vi "Pre Launch Init.vi"(11 "Nested in":refnum<class "MDI Panel Actor.lvclass">) -> (0 "error out":errorcluster, 3 "Nested out":refnum<class "MDI Panel Actor.lvclass">)   [LabVIEW 2018, in "MDI Panel Actor.lvlib" / "MDI Panel Actor.lvclass"]
uses:
  MDI Panel Actor.lvclass
  MDI Panel Actor.lvclass/MDI Panel Actor.ctl
  <vilib>/MGI/Panel Manager/Panel Actor/Panel Actor/Panel Actor.lvclass
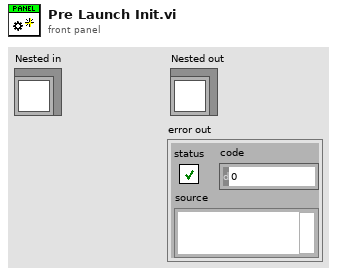
[diagram p1: front panel]
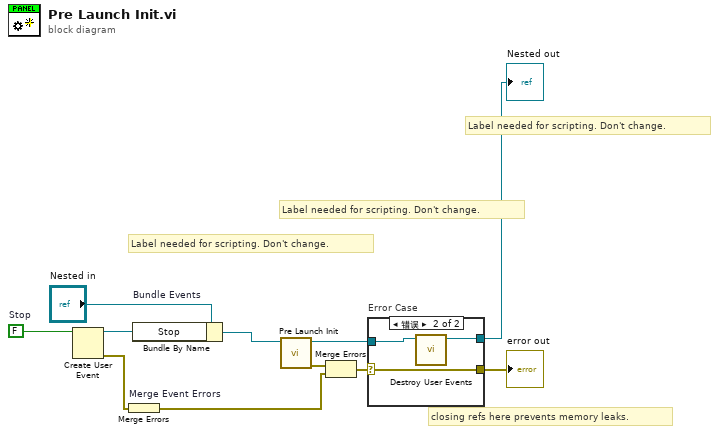
[diagram p0: block diagram]
diagram:
  w10 = FALSE  # Stop
  # "Label needed for scripting. Don't change."
  # "Label needed for scripting. Don't change."
  # "Label needed for scripting. Don't change."
  # "closing refs here prevents memory leaks."
  n1 = Create User Event(user event datatype=w10) -> (user event=w7:refnum<user-event>, error out=w9:errorcluster)  [unwired: 1 in]
  n2 = Merge Errors "Merge Event Errors"(w9) -> (w2:errorcluster)
  n3 = Bundle By Name "Bundle Events"(cluster="Nested in", "Stop"=w7) -> (w4:refnum<class "MDI Panel Actor.lvclass">)
  n4 = call-parent "Pre Launch Init.vi"("Panel Actor in"=w4) -> ("error out"=w3:errorcluster, "Panel Actor out"=w5:refnum<class "MDI Panel Actor.lvclass">)  [unwired: 9 in]
  n5 = Merge Errors ("合并错误")(w3, w2) -> (w1:errorcluster)
  n6 = case "Error Case" shown="错误" w1 {
    selector: w1 -> [w12 w16]
    tunnel: w5 -> [w13 w15]
    tunnel: [w13 w14] -> w8
    tunnel: [w12 w16] -> w6
    frame No Error {
    }
    frame Error {
      n7 = call "Destroy User Events.vi"("UI Template in"=w15) -> ("UI Template out"=w14:refnum<class "MDI Panel Actor.lvclass">)  [unwired: 10 in]
    }
  }
  "error out" <- w6
  "Nested out" <- w8
